vi "emi_Error Filter.vi"   [LabVIEW 2011]
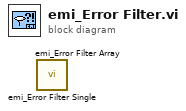
[diagram p0: block diagram]
diagram:
  n1 = call "emi_Error Filter Single.vi"() -> ()  [unwired: 14 in, 2 out]
  n2 = call "emi_Error Filter Array.vi"() -> ()  [unwired: 14 in, 2 out]
